vi "oa_Check Spectral Map Settings.vi"(6 "plot type":u16(ring) items=["Frequency-Time", "Time-Frequency", "RPM-Frequency", "Frequency-RPM", "RPM-Order", "Order-RPM"], 8 "error in (no error)":errorcluster, 9 "spectral settings":T1={"window type"=1, "number of lines"=400} {"number of lines" min=2; "window type" items=["None"=0, "Hanning"=1, "Hamming"=2, "Blackman-Harris"=3, "Exact Blackman"=4, "Blackman"=5, "Flat Top"=6, "4 Term B-Harris"=7, "7 Term B-Harris"=8, "Low Sidelobe"=9, "Gaussian"=62]}, 11 "segment":cluster{"start":dbl, "end":dbl, "step":dbl} {"step" format="%.2f"; "end" format="%.2f"; "start" format="%.2f"}) -> (0 "error out":errorcluster, 1 "spectral settings out":T1, 3 "segment out":cluster{"start":dbl, "end":dbl, "step":dbl} {"step" format="%.2f"; "end" format="%.2f"; "start" format="%.2f"}, 5 "reset":bool)   [LabVIEW 2017, in "SoundVib_Resampling.lvlib"]
uses:
  <vilib>/addons/Sound and Vibration/Order Analysis/Resample Order Tracking/SoundVib_Resampling.lvlib
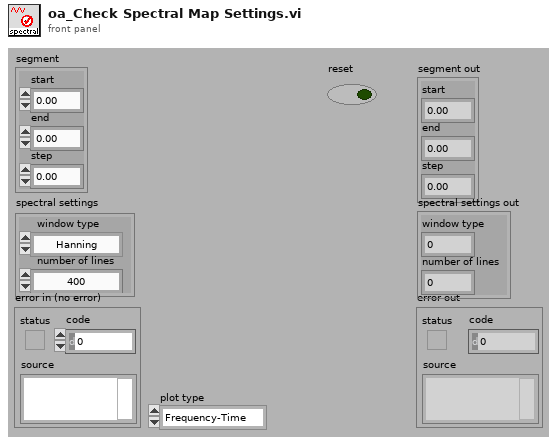
[diagram p1: front panel]
types:
  T1 = cluster{"window type":u32, "number of lines":i32}
  T2 = cluster{"start (s)":dbl, "end (s)":dbl, "step (s)":dbl}
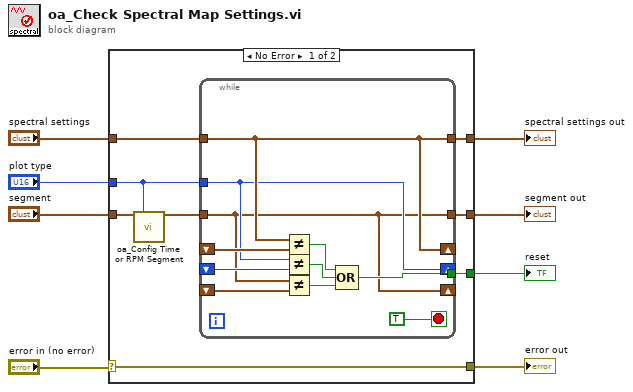
[diagram p0: block diagram]
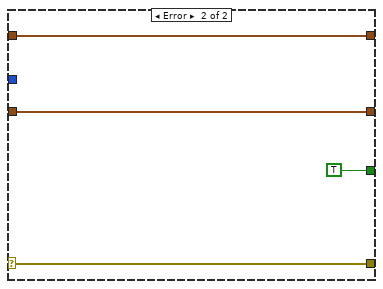
[diagram p2: hidden frame]
diagram:
  n1 = case shown="No Error" "error in (no error)" {
    selector: "error in (no error)" -> [w12 w31]
    tunnel: [w12 w31] -> w7
    tunnel: "spectral settings" -> [w16 w29]
    tunnel: "plot type" -> [w9 _]
    tunnel: [w15 w29] -> w1
    tunnel: "segment" -> [w11 w28]
    tunnel: [w14 TRUE] -> w3
    tunnel: [w13 w28] -> w2
    frame No Error {
      n2 = call <vilib>:"oa_Config Time or RPM Segment.vi"("time segment"=w11, "plot type"=w9) -> ("time segment out"=w10:T2)  [unwired: 8 in, 5 out]
      n3 = while {
        tunnel: w16 -> [w22]
        tunnel: w9 -> [w21]
        shift-right: [w22] -> _
        shift-left: _ -> [w26]
        shift-right: [w21] -> _
        shift-left: _ -> [w25]
        tunnel: [w22] -> w15
        tunnel: w10 -> [w17]
        shift-right: [w17] -> _
        shift-left: _ -> [w20]
        tunnel: [w18] -> w14
        tunnel: [w17] -> w13
        stop <- TRUE stop-if-true
        n4 = Not Equal?(x=w22, y=w26) -> (x != y?=w24:bool)
        n5 = Not Equal?(x=w21, y=w25) -> (x != y?=w23:bool)
        n6 = Not Equal?(x=w17, y=w20) -> (x != y?=w19:bool)
        n7 = Compound Arithmetic op=OR(w24, w23, w19) -> (w18:bool)
      }
    }
    frame Error {
    }
  }
  "error out" <- w7
  "segment out" <- w2
  "reset" <- w3
  "spectral settings out" <- w1
